vi "Test Map to Array.vi"(8 "error in":errorcluster) -> (0 "error out":errorcluster, 2 "passed":bool)   [LabVIEW 2020]
uses:
  2183a770-0473-3fdd-803c-8aeb4b9cb93f.vi
  source/library/Map to VArray of Clusters.vi
  source/library/Get Collection Subtype.vi
  source/library/Array of Clusters to VMap.vi
  <vilib>/addons/_JKI Toolkits/Caraya/classes/Assert/Assert True.vi
  <vilib>/addons/_JKI Toolkits/Caraya/classes/Test/Test.lvclass
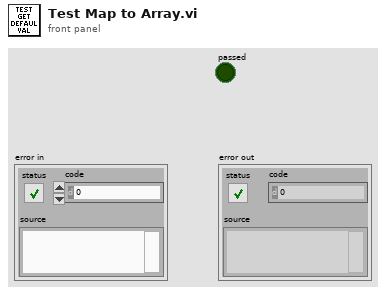
[diagram p1: front panel]
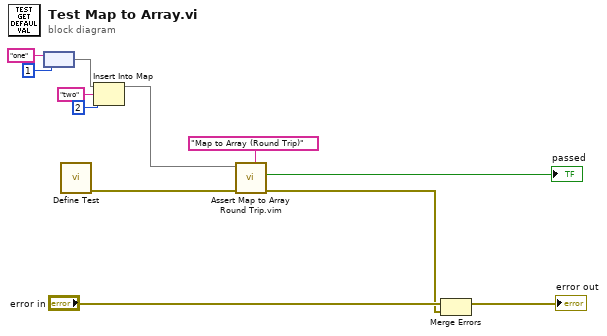
[diagram p0: block diagram]
diagram:
  n1 = node("one" ("key"), 1 ("value")) -> (w9:map{string, i32})
  n2 = call <vilib>:"Define Test.vi"() -> ("error out"=w4:errorcluster)  [unwired: 11 in]
  n3 = Insert Into Map(map in=w9, key="two", value=2) -> (map out=w2:map{string, i32})  [unwired: 2 out]
  n4 = call "Assert Map to Array Round Trip.vim"("Label"="Map to Array (Round Trip)", "error in (no error)"=w4, "Map"=w2) -> ("error out"=w10:errorcluster, "Passed"=→"passed":bool)  [unwired: 7 in]
  n5 = Merge Errors("error in", w10) -> (→"error out":errorcluster)
